vi "test输出.vi"() -> ()   [LabVIEW 2010]
panel:
  out "数值":i32
  out "关闭？":bool
  in  "停止":bool
  in  "A":i32
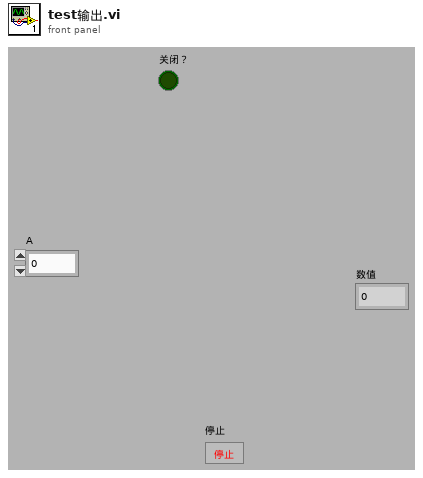
[diagram p1: front panel]
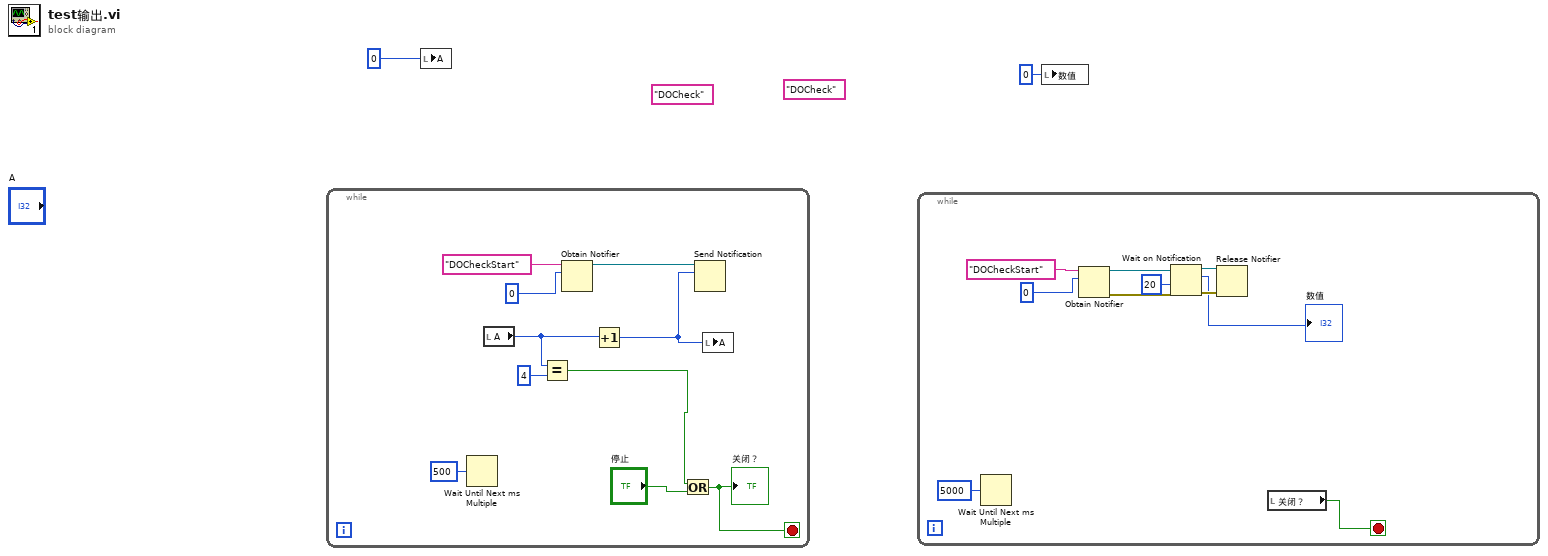
[diagram p0: block diagram]
diagram:
  (unwired) "DOCheck" ("通知")
  (unwired) "DOCheck" ("通知")
  n1 = while {
    stop <- w9 stop-if-true
    n2 = Wait Until Next ms Multiple(millisecond multiple=u32 500 ("毫秒倍数")) -> ()  [unwired: 1 out]
    n3 = local read "A"() -> (w4:i32)
    n4 = Equal?(x=w4, y=4) -> (x = y?=w11:bool)
    n5 = Obtain Notifier(name (unnamed)="DOCheckStart" ("名称（未命名）"), notification data type=0) -> (notifier out=w7:refnum<notifier>)  [unwired: 2 in, 2 out]
    n6 = Increment(x=w4) -> (x+1=w3:i32)
    n7 = Or(x=w11, y="停止") -> (x .or. y?=w9:bool)
    "关闭？" <- w9
    n8 = Send Notification(notification=w3, notifier=w7) -> ()  [unwired: 1 in, 2 out]
    n9 = local write "A"(w3) -> ()
  }
  n10 = local write "A"(0 ("A")) -> ()
  n11 = while {
    stop <- w16 stop-if-true
    n12 = Wait Until Next ms Multiple(millisecond multiple=u32 5000 ("毫秒倍数")) -> ()  [unwired: 1 out]
    n13 = Obtain Notifier(name (unnamed)="DOCheckStart" ("名称（未命名）"), notification data type=0) -> (notifier out=w18:refnum<notifier>, error out=w17:errorcluster)  [unwired: 2 in, 1 out]
    n14 = Wait on Notification(notifier=w18, timeout in ms (-1)=20 ("超时毫秒(-1)"), error in (no error)=w17) -> (notifier out=w20:refnum<notifier>, notification=→"数值":i32, error out=w21:errorcluster)  [unwired: 1 in, 1 out]
    n15 = Release Notifier(notifier=w20, error in (no error)=w21) -> ()  [unwired: 1 in, 3 out]
    n16 = local read "关闭？"() -> (w16:bool)
  }
  n17 = local write "数值"(0 ("数值")) -> ()
